vi "StateMachine.vi"() -> ()   [LabVIEW 2014]
uses:
  Control 3.ctl
panel:
  in  "Menu":T1
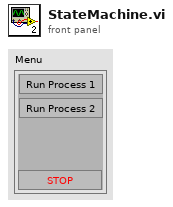
[diagram p1: front panel]
types:
  T1 = cluster{"Process 1":bool, "Process 2":bool, bool}
  T2 = typedef "Control 3.ctl" = enum32{"Idle", "Process 1", "Process 2", "Stop"}
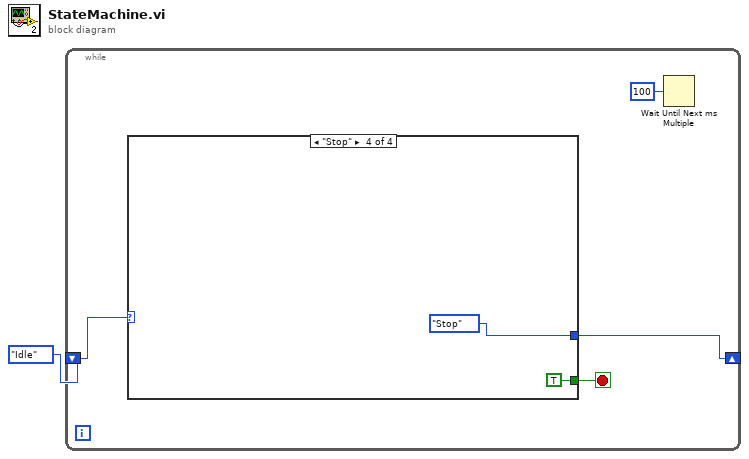
[diagram p0: block diagram]
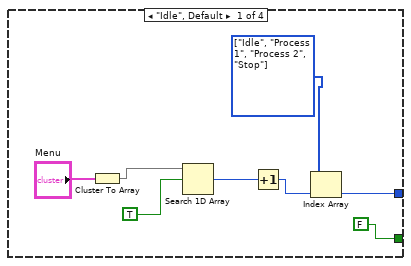
[diagram p2: hidden frame]
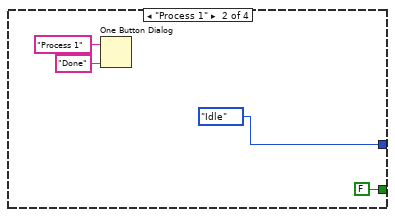
[diagram p3: hidden frame]
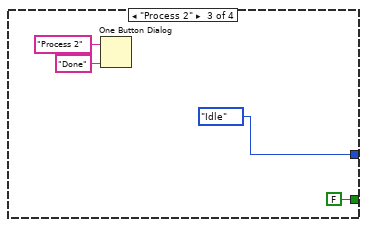
[diagram p4: hidden frame]
diagram:
  n1 = while {
    shift-right: [w2] -> _
    shift-left: Control_3."Idle" ("State Enum") -> [w5]
    stop <- w4 stop-if-true
    n2 = case shown="\"Stop\"" w5 {
      tunnel: [FALSE FALSE FALSE TRUE] -> w4
      tunnel: [w6 Control_3."Idle" ("State Enum") Control_3."Idle" ("State Enum") Control_3."Stop" ("State Enum")] -> w2
      frame "Idle", Default {
        w8 = T2[] [enum."Idle", enum."Process 1", enum."Process 2", enum."Stop"] items=["Idle", "Process 1", "Process 2", "Stop"] ("array")
        n3 = Cluster To Array(cluster="Menu") -> (array=w12:bool[])
        n4 = Search 1D Array(1D array=w12, element=TRUE) -> (index of element=w10:i32)  [unwired: 1 in]
        n5 = Increment(x=w10) -> (x+1=w9:i32)
        n6 = Index Array(array=w8, index=w9) -> (element=w6:T2)
      }
      frame "Process 1" {
        n7 = One Button Dialog(message="Process 1", button name ("OK")="Done") -> ()  [unwired: 1 out]
      }
      frame "Process 2" {
        n8 = One Button Dialog(message="Process 2", button name ("OK")="Done") -> ()  [unwired: 1 out]
      }
      frame "Stop" {
      }
    }
    n9 = Wait Until Next ms Multiple(millisecond multiple=u32 100) -> ()  [unwired: 1 out]
  }
